vi "Operation.vi"() -> (3 "Out Operation":refnum<class "Operation.lvclass">)   [LabVIEW 2024, in "Operation.lvclass"]
uses:
  Operation.lvclass
  Operation.lvclass/Operation.ctl
panel:
  in  "Operation.lvclass":refnum<class "Operation.lvclass">
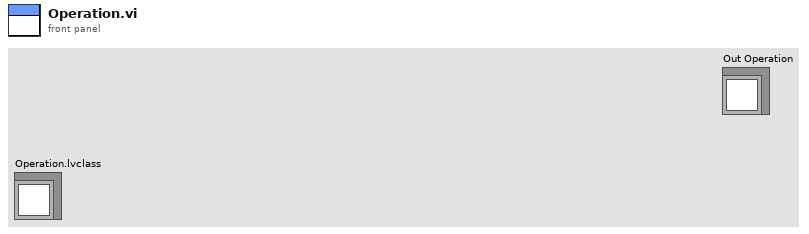
[diagram p1: front panel]
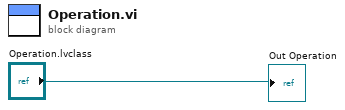
[diagram p0: block diagram]
diagram:
  "Out Operation" <- "Operation.lvclass"
